vi "dfd_Super Narrowband Filter Design Convert to New Type.vi"(7 "new filter type":T1(ring), 8 "ripple specs":T2={"passband"=0.0, "stopband"=0.0, "dB/linear? (T: dB)"=TRUE}, 10 "fstop":dbl, 11 "fpass":dbl) -> (0 "ripple specs out":T2={"passband"=0.0, "stopband"=0.0, "dB/linear? (T: dB)"=TRUE}, 2 "fstop out":dbl, 3 "fpass out":dbl)   [LabVIEW 2017, in "NI_DigFilter_Process.lvlib"]
doc: "Converts the filter specification according the type of narrowband filter."
uses:
  <vilib>/addons/Digital Filter Design/NI_DigFilter_Process.lvlib
  <vilib>/addons/Digital Filter Design/_Objects.llb/DFD Filter Ripple Specification (Design).ctl
  <vilib>/addons/Digital Filter Design/NI_DigFilterLicensed.lvlib
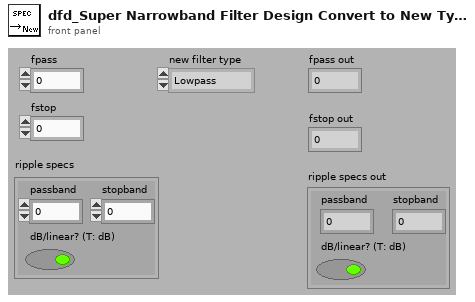
[diagram p1: front panel]
types:
  T1 = enum32{"Lowpass", "Highpass", "Bandpass", "Bandstop", "Wideband-Lowpass", "Wideband-Highpass"}
  T2 = typedef "NI_DigFilterLicensed.lvlib/DFD Filter Ripple Specification (Design).ctl" = cluster{"passband":dbl, "stopband":dbl, "dB/linear? (T: dB)":bool}
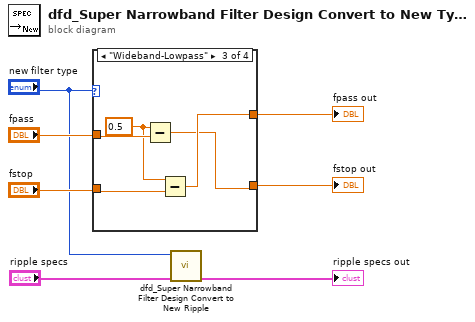
[diagram p0: block diagram]
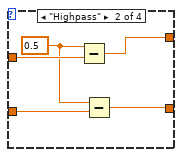
[diagram p3: hidden frame]
diagram:
  n1 = case shown="\"Wideband-Lowpass\"" "new filter type" {
    tunnel: "fpass" -> [w9 w12 w18 w20]
    tunnel: "fstop" -> [w8 w11 w19 w21]
    tunnel: [w9 w14 w16 w21] -> w4
    tunnel: [w8 w13 w15 w20] -> w5
    frame "Lowpass", Default {
    }
    frame "Highpass" {
      w10 = 0.5 ("x")
      n2 = Subtract(x=w10, y=w12) -> (x-y=w14:dbl)
      n3 = Subtract(x=w10, y=w11) -> (x-y=w13:dbl)
    }
    frame "Wideband-Lowpass" {
      w17 = 0.5 ("x")
      n4 = Subtract(x=w17, y=w18) -> (x-y=w15:dbl)
      n5 = Subtract(x=w17, y=w19) -> (x-y=w16:dbl)
    }
    frame "Wideband-Highpass" {
    }
  }
  "fpass out" <- w4
  "fstop out" <- w5
  n6 = call <vilib>:"dfd_Super Narrowband Filter Design Convert to New Ripple.vi"("ripple specs in"="ripple specs", "new filter type"="new filter type") -> ("ripple specs out"=→"ripple specs out":T2)  [unwired: 9 out]
